vi "Calculate Gyro.vi"(8 "Field Oriented Control?":bool, 11 "Yaw":dbl) -> (3 "Gyro Angle":dbl)   [LabVIEW 2020]
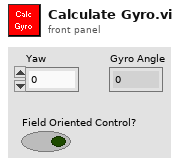
[diagram p1: front panel]
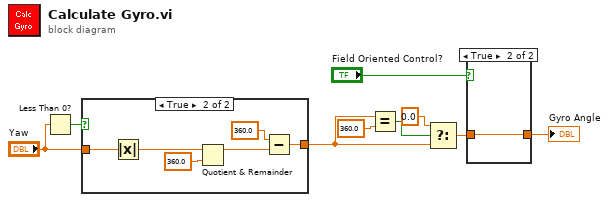
[diagram p0: block diagram]
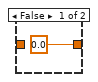
[diagram p2: hidden frame]
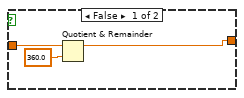
[diagram p3: hidden frame]
diagram:
  n1 = Less Than 0?(x="Yaw") -> (x < 0?=w7:bool)
  n2 = case shown="True" w7 {
    tunnel: "Yaw" -> [w12 w17]
    tunnel: [w10 w14] -> w4
    frame False {
      n3 = Quotient & Remainder(x=w12, y=360.0) -> (x-y*floor(x/y)=w10:dbl)  [unwired: 1 out]
    }
    frame True {
      n4 = Absolute Value(x=w17) -> (abs(x)=w18:dbl)
      n5 = Quotient & Remainder(x=w18, y=360.0) -> (x-y*floor(x/y)=w15:dbl)  [unwired: 1 out]
      n6 = Subtract(x=360.0, y=w15) -> (x-y=w14:dbl)
    }
  }
  n7 = Equal?(x=w4, y=360.0) -> (x = y?=w6:bool)
  n8 = Select(t=0.0, s=w6, f=w4) -> (s? t:f=w3:dbl)
  n9 = case shown="True" "Field Oriented Control?" {
    tunnel: [0.0 w20] -> w1
    tunnel: w3 -> [_ w20]
    frame False {
    }
    frame True {
    }
  }
  "Gyro Angle" <- w1
